vi "Launch Data Logger.vi"(8 "error in":errorcluster, 11 "Series Actor in":refnum<class "Series Actor.lvclass">) -> (0 "error out":errorcluster, 3 "Series Actor out":refnum<class "Series Actor.lvclass">)   [LabVIEW 2023, in "Series Actor.lvlib" / "Series Actor.lvclass"]
uses:
  Series Actor.lvclass
  Series Actor.lvclass/Series Actor.ctl
  Data Logger Actor/Data Logger Actor/Data Logger Actor/Data Logger Actor.lvclass
  6f6e41d2-7b58-4c34-926f-9e220067dc52.vi
  6f6e41d2-7b58-4c34-926f-9e220067dc52.vi/a4169a97-72fc-4003-a778-603cf20cafa0.vi
  <vilib>/JDP Science/JSONtext/Find Item.vi
  <vilib>/JDP Science/JSONtext/Next JSON Value.vi
  <vilib>/JDP Science/JSONtext/String Subset.vi
  <vilib>/JDP Science/JSONtext/Parsing/Advance past next JSON Value (inlined COPY).vi
  <vilib>/JDP Science/JSONtext/Parsing/Advance past whitespace.vi
  <vilib>/JDP Science/JSONtext/Parsing/Advance past String.vi
  <vilib>/JDP Science/JSONtext/Parsing/Advance past Number.vi
  <vilib>/JDP Science/JSONtext/Parsing/Advance past Line Ending.vi
  <vilib>/MGI/Panel Manager/Panel/Panel/Subpanel/Subpanel.lvclass
  <vilib>/JDP Science/JSONtext/Parsing/Parse Full Path or Item Name.vi
  <vilib>/JDP Science/JSONtext/Parsing/Advance past Array.vi
  <vilib>/JDP Science/JSONtext/Parsing/Advance past Object.vi
  <vilib>/JDP Science/JSONtext/support/Error Cluster From Code.vi
  <vilib>/JDP Science/JSONtext/Offset/Find Item Locations by Path.vi
  <vilib>/JDP Science/JSONtext/JSON text to Variant.vi
  <vilib>/Utility/error.llb/Error Cluster From Error Code.vi
  <vilib>/MGI/Panel Manager/Panel/Panel/Subpanel/Subpanel.vi
  <vilib>/JDP Science/JSONtext/LVClass Serializer/JSONtext LVClass Serializer.lvclass
  <vilib>/MGI/Panel Manager/Panel Actor/Panel Actor/Panel Actor.lvclass
  <vilib>/MGI/Panel Manager/Panel/Panel.lvlib
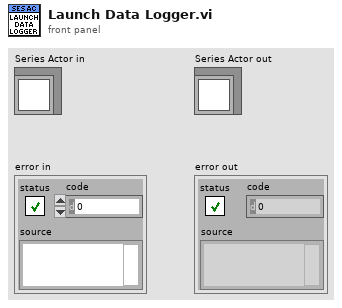
[diagram p1: front panel]
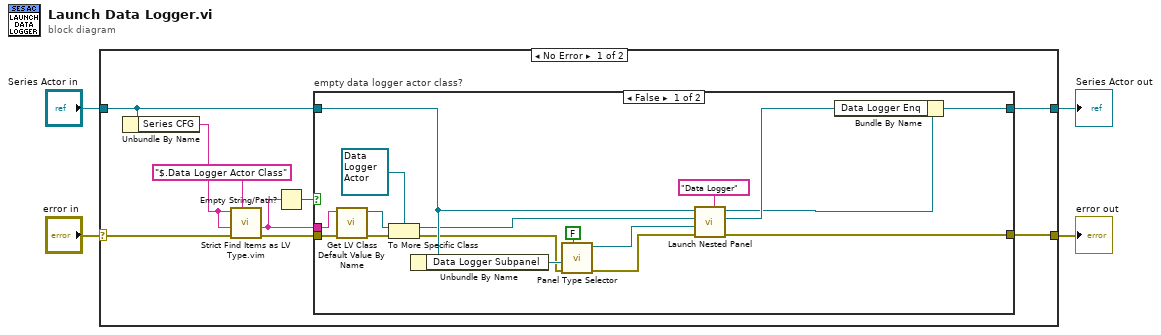
[diagram p0: block diagram]
diagram:
  n1 = case shown="No Error" "error in" {
    selector: "error in" -> [w13 w34]
    tunnel: [w7 w34] -> w3
    tunnel: [w9 w33] -> w1
    tunnel: "Series Actor in" -> [w8 w33]
    frame No Error {
      n2 = Unbundle By Name(w8) -> ("Series CFG"=w11:string)
      n3 = call "Strict Find Items as LV Type.vim"("$Path or Item Name"="$.Data Logger Actor Class", "error in"=w13, "Data Type and Default Value"=w11, "JSON"=w11) -> ("error out"=w10:errorcluster, "Data out"=w5:string)  [unwired: 6 in]
      n4 = Empty String/Path?(string/path=w5) -> (empty?=w6:bool)
      n5 = case "empty data logger actor class?" shown="False" w6 {
        tunnel: w10 -> [w30 w32]
        tunnel: [w27 w31] -> w9
        tunnel: w8 -> [w26 w31]
        tunnel: [w23 w32] -> w7
        tunnel: w5 -> [w22 _]
        frame False {
          n6 = call <vilib>:"Get LV Class Default Value By Name.vi"("error in (no error)"=w30, "class name"=w22) -> ("error out"=w29:errorcluster, "object"=w28:refnum<class>)  [unwired: 8 in]
          n7 = To More Specific Class(target class=refnum<class "Data Logger Actor.lvclass"> refnum ("Data Logger Actor.lvlib:Data Logger Actor.lvclass"), reference=w28, error in=w29) -> (specific class reference=w20:refnum<class "Data Logger Actor.lvclass">, error out=w16:errorcluster)
          n8 = Unbundle By Name(w26) -> ("Data Logger Subpanel"=w18:refnum<vi>)
          n9 = call-poly <vilib>:"Panel Type Selector.vi"("Autoshow? (T)"=FALSE, "Error In"=w16, "Sub Panel"=w18) -> ("Error Out"=w17:errorcluster, "Subpanel Out"=w14:refnum<class "Subpanel.lvclass">)  [unwired: 7 in]
          n10 = call <vilib>:"Launch Nested Panel.vi"("Debug Alias"="Data Logger", "error in (no error)"=w17, "Panel"=w14, "Nested Panel Actor"=w20, "Panel Actor in"=w26) -> ("error out"=w23:errorcluster, "Nested Actor's Enqueuer"=w25:refnum<class "Message Enqueuer.lvclass">, "Panel Actor out"=w24:refnum<class "Series Actor.lvclass">)  [unwired: 3 in, 1 out]
          n11 = Bundle By Name(cluster=w24, "Data Logger Enq"=w25) -> (w27:refnum<class "Series Actor.lvclass">)
        }
        frame True {
        }
      }
    }
    frame Error {
    }
  }
  "error out" <- w3
  "Series Actor out" <- w1
